vi "HTTP Get.vi"(8 "error in (no error)":errorcluster caption="错误输入（无错误）", 11 "url":string) -> (0 "error out":errorcluster caption="错误输出")   [LabVIEW 2016, in "Bark.lvlib" / "Bark.lvclass"]
uses:
  Bark.lvclass
  <vilib>/httpClient/LabVIEWHTTPClient.lvlib
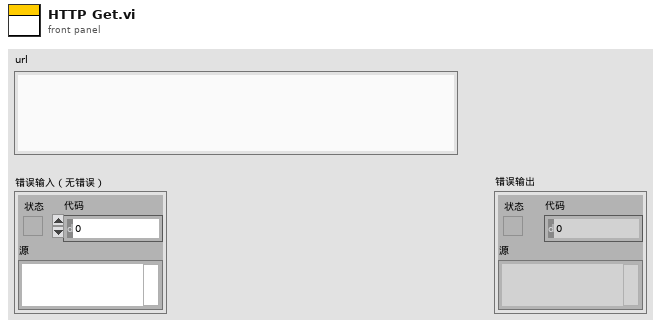
[diagram p1: front panel]
types:
  T1 = typedef "LabVIEWHTTPClient.lvlib/ClientHandle.ctl" = refnum<k1>
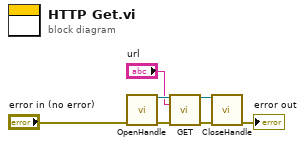
[diagram p0: block diagram]
diagram:
  n1 = call <vilib>:"OpenHandle.vi"("error in (no error)"="error in (no error)") -> ("client handle out"=w7:T1, "error out"=w6:errorcluster)  [unwired: 13 in]
  n2 = call <vilib>:"GET.vi"("client handle"=w7, "url"="url", "error in (no error)"=w6) -> ("client handle out"=w5:T1, "error out"=w4:errorcluster)  [unwired: 9 in, 2 out]
  n3 = call <vilib>:"CloseHandle.vi"("client handle"=w5, "error in (no error)"=w4) -> ("error out"=→"error out":errorcluster)  [unwired: 13 in]
